vi "Set-Settings-notif.vi"(8 "error in (no error)":errorcluster, 10 "Settings source":T1, 11 "UI ref. in":refnum<data-value>) -> (0 "error out":errorcluster, 3 "UI ref.":refnum<data-value>)   [LabVIEW 2013, in "CameraVision.lvlib" / "CV-UI.lvclass"]
uses:
  CV-UI.lvclass
  Settings-source.ctl
  CV-UI.lvclass/CV-UI.ctl
  Read Settings-source.vi
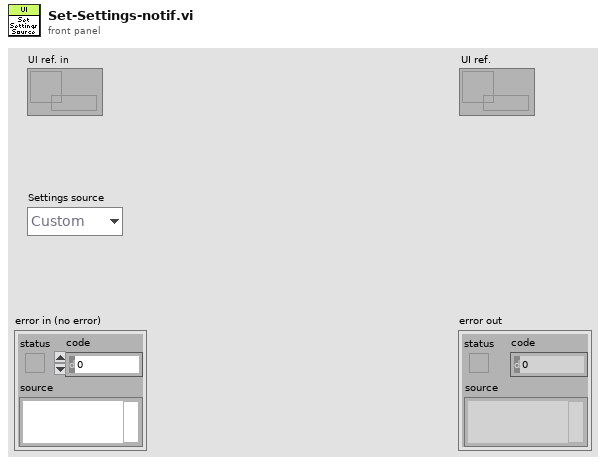
[diagram p1: front panel]
types:
  T1 = typedef "CameraVision.lvlib/CV-UI.lvclass/Settings-source.ctl" = enum16{"Custom", "Default", "Last used", "File"}
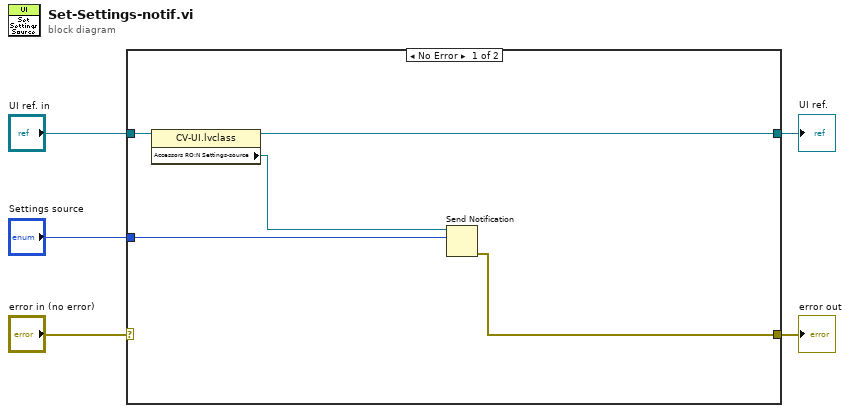
[diagram p0: block diagram]
diagram:
  n1 = case shown="No Error" "error in (no error)" {
    selector: "error in (no error)" -> [_ w12]
    tunnel: [w7 w12] -> w4
    tunnel: "UI ref. in" -> [w9 w11]
    tunnel: [w8 w11] -> w2
    tunnel: "Settings source" -> [w10 _]
    frame No Error {
      n2 = property class="CV-UI.lvclass"(reference=w9) -> (reference out=w8:refnum<data-value>, "Accessors RO:N Settings-source"=w6:refnum<notifier>)  [unwired: 1 in, 1 out]
      n3 = Send Notification(notification=w10, notifier=w6) -> (error out=w7:errorcluster)  [unwired: 1 in, 1 out]
    }
    frame Error {
    }
  }
  "error out" <- w4
  "UI ref." <- w2
